vi "NI VeriStand - Get System State.vi"(8 "error in (no error)":errorcluster, 11 "WorkspaceManager in":T2) -> (0 "error out":errorcluster, 1 "Targets":string[](array[string]), 2 "System State":T1 items=["Idle", "Active"], 3 "WorkspaceManager  out":T2, 5 "System Definition File":path)   [LabVIEW 2020, in "NI_VS Workspace ExecutionAPI.lvlib"]
doc: "Gets the current state of the system to which the VeriStand Gateway is connected."
uses:
  <vilib>/NI VeriStand/Execution/Workspace/NI_VS Workspace ExecutionAPI.lvlib
  <vilib>/NI VeriStand/Execution/Workspace/WorkspaceAPI.ctl
  NationalInstruments.VeriStand.ClientAPI
  <vilib>/NI VeriStand/Execution/Workspace/SystemState.ctl
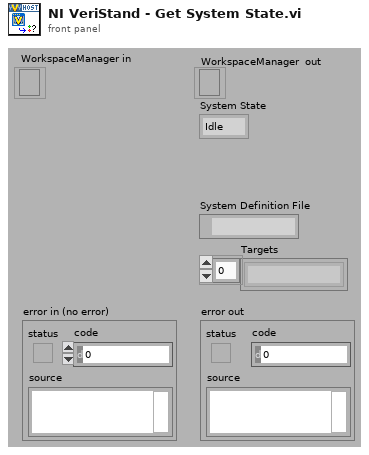
[diagram p1: front panel]
types:
  T1 = typedef "NI_VS Workspace ExecutionAPI.lvlib/SystemState.ctl" = u8
  T2 = typedef "NI_VS Workspace ExecutionAPI.lvlib/WorkspaceAPI.ctl" = refnum<k24>
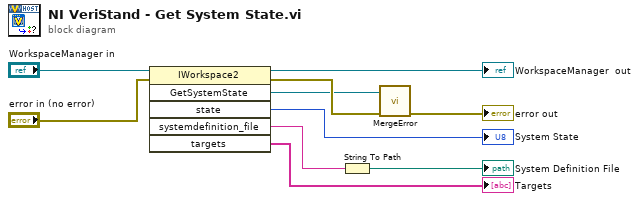
[diagram p0: block diagram]
diagram:
  n1 = invoke class="IWorkspace2" method="GetSystemState"(reference="WorkspaceManager in", error in="error in (no error)") -> (reference out=→"WorkspaceManager  out":T2, error out=w8:errorcluster, "GetSystemState"=w7:refnum<k24>, "state"=→"System State":u8, "systemdefinition_file"=w2:string, "targets"=→"Targets":string[])  [unwired: 4 in]
  n2 = String To Path(string=w2) -> (path=→"System Definition File":path)
  n3 = call <vilib>:"MergeError.vi"("error in (no error)"=w8, "Error"=w7) -> ("error out"=→"error out":errorcluster)  [unwired: 9 out]
